vi "BriqueISOSPI.vi"(8 "errin":errorcluster, 10 "nbmodule":i32=8, 11 "visain":refnum<visa-resource-name>) -> (0 "errout":errorcluster, 1 "chaîne résultante":string, 2 "NTC Temperatures":string[][](table), 3 "Cell Voltages":string[][](table), 4 "TCellmax":dbl, 5 "VCellmax":dbl, 6 "TCellmin":dbl, 7 "VCellmin":dbl)   [LabVIEW 2020]
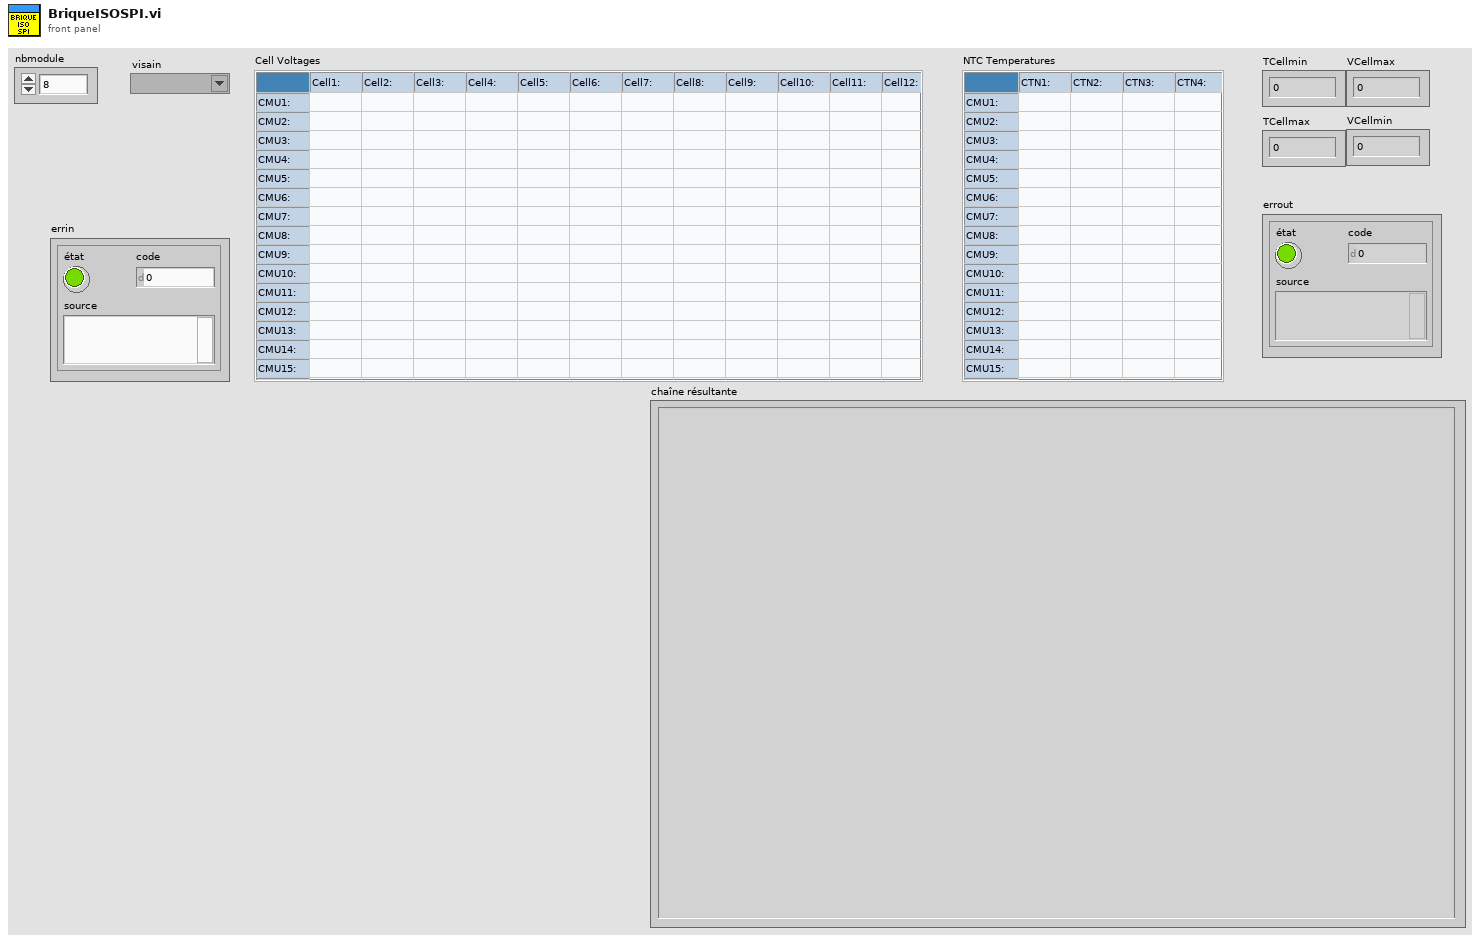
[diagram p1: front panel]
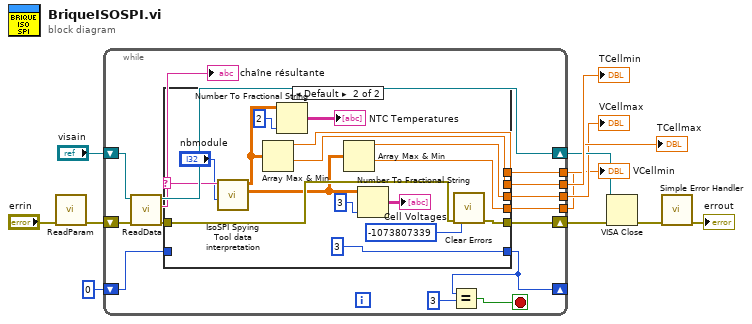
[diagram p0: block diagram]
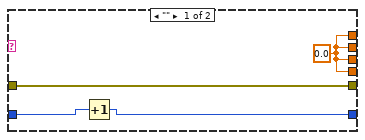
[diagram p2: hidden frame]
diagram:
  n1 = call "ReadParam.vi"("error in (no error)"="errin") -> ("error out"=w1:errorcluster)  [unwired: 10 in]
  n2 = while {
    shift-right: [w26] -> w7
    shift-left: "visain" -> [w25]
    shift-right: [w19] -> w8
    shift-left: w1 -> [w18]
    tunnel: [w23] -> w5
    tunnel: [w22] -> w4
    tunnel: [w21] -> w11
    tunnel: [w20] -> w12
    shift-right: [w14] -> _
    shift-left: 0 ("x") -> [w16]
    stop <- w24 stop-if-true
    n3 = call "ReadData.vi"("errin"=w18, "visain"=w25) -> ("errout"=w17:errorcluster, "VResult"=w13:string, "visaout"=w26:refnum<visa-resource-name>)  [unwired: 6 in, 1 out]
    "chaîne résultante" <- w13
    n4 = case shown="Default" w13 {
      selector: w13 -> [_ w33]
      tunnel: [w30 w46] -> w23
      tunnel: [w30 w45] -> w22
      tunnel: [w30 w44] -> w21
      tunnel: [w30 w43] -> w20
      tunnel: [w29 w36] -> w19
      tunnel: w17 -> [w29 w35]
      tunnel: w16 -> [w28 _]
      tunnel: [w27 3] -> w14
      frame "" {
        w30 = 0.0
        n5 = Increment(x=w28) -> (x+1=w27:i32)
      }
      frame Default {
        n6 = call "IsoSPI Spying Tool data interpretation.vi"("nbmodule"="nbmodule", "VCell"=w33) -> ("Vcell"=w32:dbl[][], "TCELL"=w40:dbl[][])  [unwired: 8 in]
        n7 = Array Max & Min(array=w40) -> (max value=w44:dbl, min value=w43:dbl)  [unwired: 2 out]
        n8 = Number To Fractional String ("Nombre en chaîne fractionnaire")(number=w40, precision (6)=i16 2 ("précision (6)")) -> (F-format string=→"NTC Temperatures":string[][])  [unwired: 2 in]
        n9 = Array Max & Min(array=w32) -> (max value=w46:dbl, min value=w45:dbl)  [unwired: 2 out]
        n10 = Number To Fractional String ("Nombre en chaîne fractionnaire")(number=w32, precision (6)=i16 3 ("précision (6)")) -> (F-format string=→"Cell Voltages":string[][])  [unwired: 2 in]
        n11 = call <vilib>:"Clear Errors.vi"("error in (no error)"=w35, "specific error code to clear (0: all)"=-1073807339) -> ("error out"=w36:errorcluster)  [unwired: 4 in, 1 out]
      }
    }
    n12 = Equal? ("Égaux ?")(x=w14, y=3) -> (x = y?=w24:bool)
  }
  "TCellmin" <- w12
  "TCellmax" <- w11
  "VCellmin" <- w4
  "VCellmax" <- w5
  n13 = VISA Close(VISA resource name=w7, error in (no error)=w8) -> (error out=w6:errorcluster)
  n14 = call <vilib>:"Simple Error Handler.vi"("error in (no error)"=w6) -> ("error out"=→"errout":errorcluster)  [unwired: 4 in, 4 out]
